vi "Get Configuration ID.vi"(8 "error in (no error)":errorcluster, 11 "Item Ref in":T1 format="%.0x") -> (0 "error out":errorcluster, 2 "Configuration ID":i32, 3 "Item Ref out":T1 format="%.0x")   [LabVIEW 2017, in "DSF System Explorer.lvlib"]
uses:
  DSF System Explorer.lvlib
  <vilib>/NI Veristand/Custom Device API/Custom Device Item Ref.ctl
  <vilib>/NI Veristand/Custom Device API/Get Item Property (I32).vi
  <vilib>/NI Veristand/Custom Device API/Custom Device API.lvlib
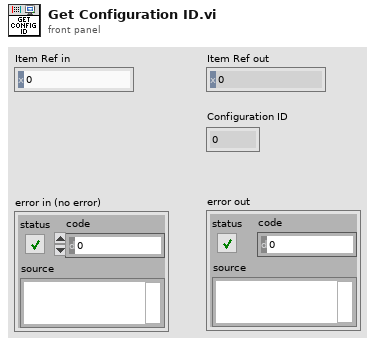
[diagram p1: front panel]
types:
  T1 = typedef "Custom Device API.lvlib/Custom Device Item Ref.ctl" = u64
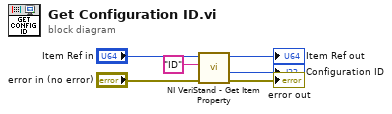
[diagram p0: block diagram]
diagram:
  n1 = call-poly <vilib>:"NI VeriStand - Get Item Property.vi"("error in (no error)"="error in (no error)", "Property Name"="ID", "Item Ref in"="Item Ref in") -> ("error out"=→"error out":errorcluster, "Value"=→"Configuration ID":i32, "Item Ref out"=→"Item Ref out":T1)  [unwired: 5 in, 1 out]
